vi "Read Analogue.vi"(8 "error in (no error)":errorcluster, 11 "Sim DMM in":refnum<class "Sim DMM.lvclass">) -> (0 "error out":errorcluster, 2 "Measurement":dbl format="%.5f", 3 "Sim DMM out":refnum<class "Sim DMM.lvclass">)   [LabVIEW 2019, in "Concrete.lvlib" / "Sim DMM.lvclass"]
uses:
  Sim DMM.lvclass
  <vilib>/numeric/Random Number (Range) DBL.vi
  Harware Abstraction/MultiIO/MIO.lvclass
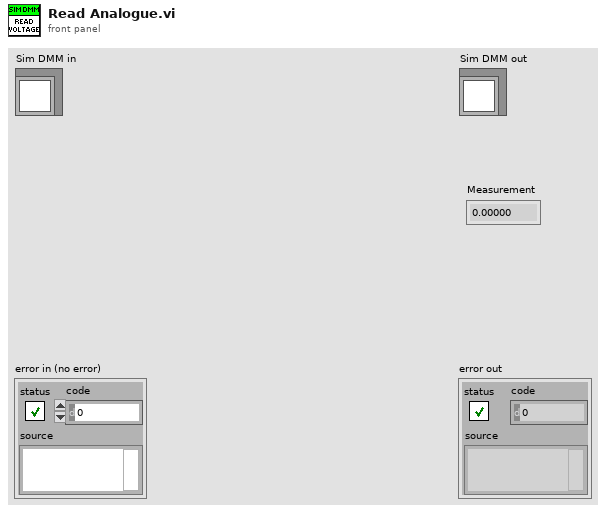
[diagram p1: front panel]
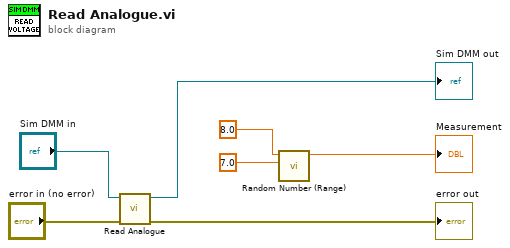
[diagram p0: block diagram]
diagram:
  n1 = call-parent "Read Analogue.vi"("error in (no error)"="error in (no error)", "DMM in"="Sim DMM in") -> ("error out"=→"error out":errorcluster, "DMM out"=→"Sim DMM out":refnum<class "Sim DMM.lvclass">)  [unwired: 7 in, 1 out]
  n2 = call-poly <vilib>:"Random Number (Range).vi"("lower bound (0)"=7.0, "upper bound (100)"=8.0) -> ("number"=→"Measurement":dbl)  [unwired: 9 in]
